vi "write_resistances_array_to_probe.vi"(8 "error in (no error)":errorcluster, 10 "resistances array":dbl[](array[numeric]), 11 "TempProbe in":refnum<class "TempProbe.lvclass">) -> (0 "error out":errorcluster, 3 "TempProbe out":refnum<class "TempProbe.lvclass">)   [LabVIEW 2010, in "TempProbe.lvclass"]
uses:
  TempProbe.lvclass
  TempProbe.lvclass/TempProbe.ctl
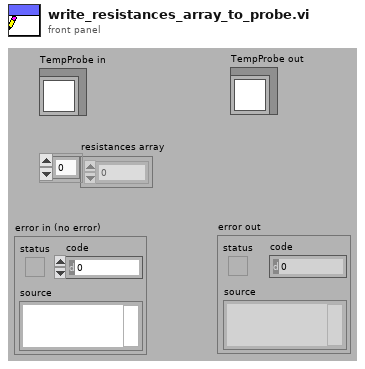
[diagram p1: front panel]
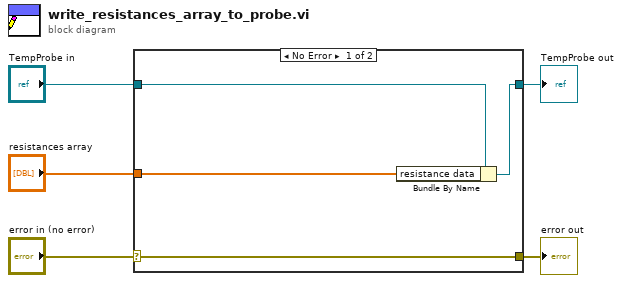
[diagram p0: block diagram]
diagram:
  n1 = case shown="No Error" "error in (no error)" {
    selector: "error in (no error)" -> [w9 w10]
    tunnel: [w9 w10] -> w4
    tunnel: [w7 w11] -> w2
    tunnel: "TempProbe in" -> [w8 w11]
    tunnel: "resistances array" -> [w6 _]
    frame No Error {
      n2 = Bundle By Name(cluster=w8, "resistance data"=w6) -> (w7:refnum<class "TempProbe.lvclass">)
    }
    frame Error {
    }
  }
  "error out" <- w4
  "TempProbe out" <- w2
